vi "Adquisicion Sonido Continuo.vi"() -> ()   [LabVIEW 2023]
uses:
  <vilib>/sound2/lvsound2.llb/Sound Data Format.ctl
  <vilib>/sound2/lvsound2.llb/Sampling Mode.ctl
  <vilib>/sound2/lvsound2.llb/Sound Input Read (DBL).vi
  <vilib>/express/express analysis/Spectral/Block/exnSpectralBlock spectral measurements power poly.vi
  <vilib>/express/express analysis/Spectral/Block/exnSpectralBlock spectral measurements power array WFM.vi
  <vilib>/express/express analysis/Spectral/XNode/ExpressSpectralMeasurementsBlockNode.xnode
  <vilib>/measure/NI_MABase.lvlib
panel:
  in  "frequency":dbl=10.0 format="%0.2p"
  in  "signal type 2":T1(ring)
  in  "offset 2":dbl format="%0.2p"
  in  "phase 2":dbl format="%.2p"
  in  "amplitude 2":dbl=1.0 format="%0.2p"
  in  "signal type":T1(ring)
  in  "offset":dbl format="%0.2p"
  in  "phase":dbl format="%.2p"
  in  "amplitude":dbl=1.0 format="%0.2p"
  out "Max banda 2":i32
  out "Max banda 1":i32
  out "XY Graph":cluster{"Array":dbl[], "Array":dbl[]}(graph)
  out "Tamaño banda 2":i32
  out "Plano Y":dbl[](array[numeric])
  out "Tamaño banda 1":i32
  out "Plano X":dbl[](array[numeric])
  in  "banda 2":dbl
  in  "banda 1":dbl
  out "Tamaño Señal":i32
  out "Espectro Señal":cluster{"f0":dbl, "df":dbl, "magnitude":dbl[]}[](graph)
  in  "stop":bool
  in  "Tiempo de refresco":dbl
  out "Señal Adquirida":waveform(dbl)[](graph)
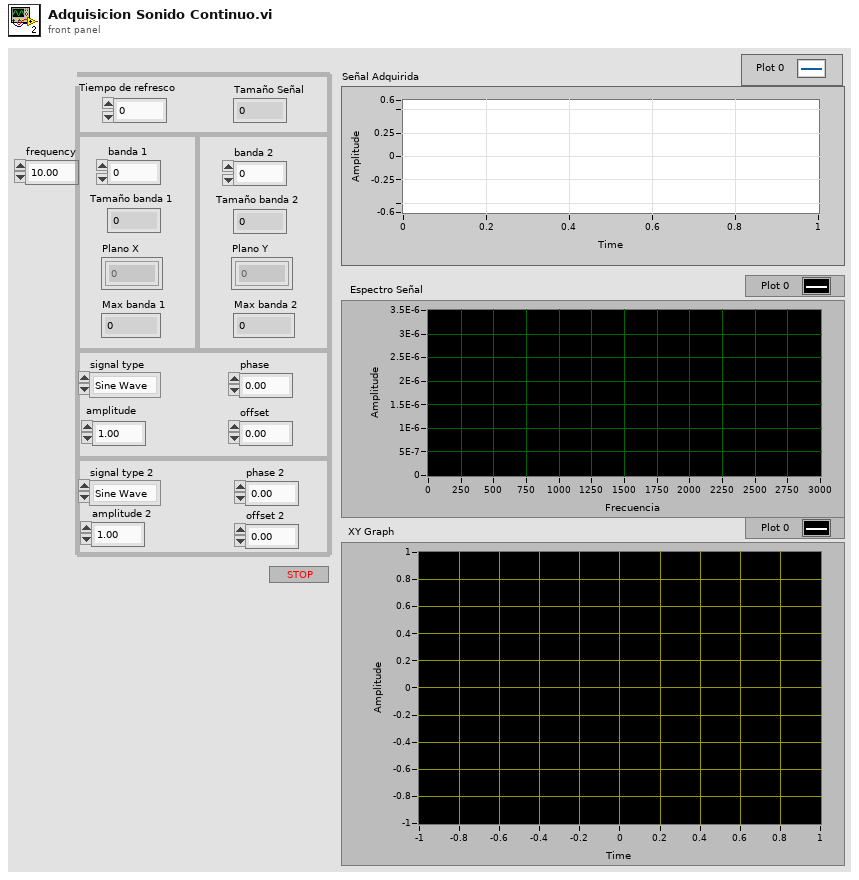
[diagram p1: front panel]
types:
  T1 = enum16{"Sine Wave", "Triangle Wave", "Square Wave", "Sawtooth Wave"}
  T2 = typedef "Sampling Mode.ctl" = i32
  T3 = typedef "Sound Data Format.ctl" = cluster{"sample rate (S/s)":dbl, "number of channels":i32, "bits per sample":i32}
  T4 = typedef "Sound Input Task ID.ctl" = u32
  T5 = cluster{"averaging mode":u16, "weighting mode":u16, "number of averages":u32}
  T6 = cluster{"dB On (F)":bool, "unwrap phase (F)":bool, "convert to degree (F)":bool}
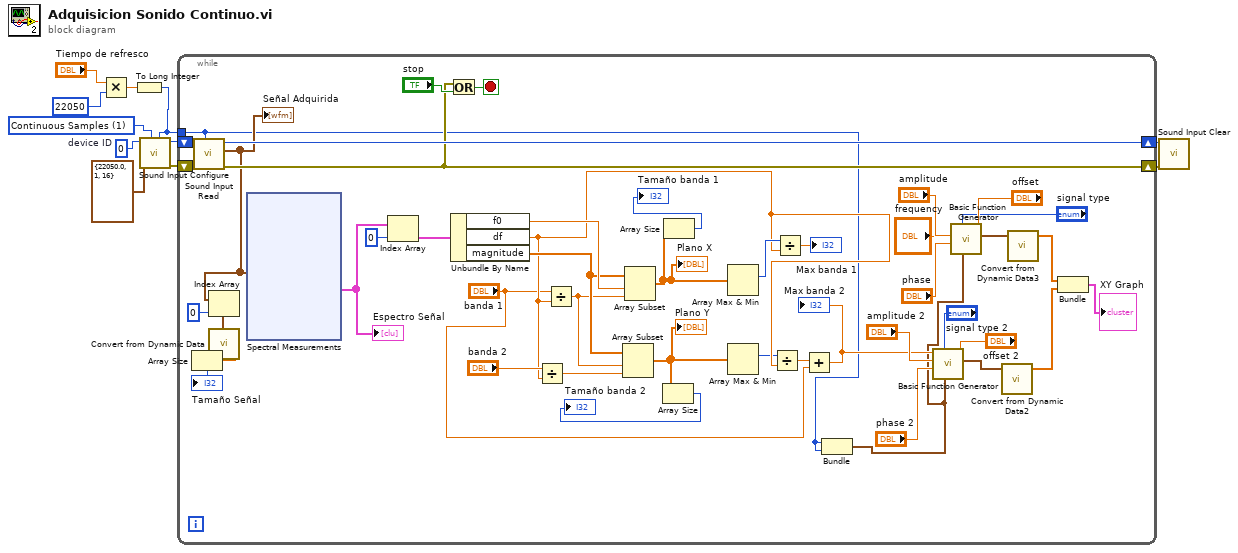
[diagram p0: block diagram]
diagram:
  w6 = u32 0  # device ID
  w10 = T2 1 items=["Finite Samples", "Continuous Samples"] ("sample mode")
  n1 = Multiply(x="Tiempo de refresco", y=22050 ("number of samples/ch")) -> (x*y=w5:dbl)
  n2 = To Long Integer(number=w5) -> (32bit integer=w7:i32)
  n3 = call <vilib>:"Sound Input Configure.vi"("number of samples/ch"=w7, "sample mode"=w10, "sound format"=T3 {"sample rate (S/s)"=22050.0, "number of channels"=1, "bits per sample"=16}, "device ID"=w6) -> ("error out"=w8:errorcluster, "task ID"=w9:T4)  [unwired: 6 in]
  n4 = while {
    tunnel: w7 -> [w12]
    shift-right: [w53] -> w3
    shift-left: w9 -> [w57]
    shift-right: [w52] -> w2
    shift-left: w8 -> [w56]
    stop <- w54 stop-if-true
    n5 = call-poly <vilib>:"Sound Input Read.vi"("number of samples/ch"=w12, "error in (no error)"=w56, "task ID"=w57) -> ("error out"=w52:errorcluster, "data"=w49:waveform(dbl)[], "task ID out"=w53:T4)  [unwired: 6 in]
    "Señal Adquirida" <- w49
    n6 = Index Array(array=w49, index=0) -> (element=w47:waveform(dbl))
    n7 = call "Convert from Dynamic Data"("Dynamic Data Type"=w47) -> ("Array"=w46:dbl[])  [unwired: 3 in]
    n8 = Array Size(array=w46) -> (size(s)=→"Tamaño Señal":i32)
    n9 = xnode "Spectral Measurements"("Signals"=w49) -> ("Power Spectrum"=w51:cluster{"f0":dbl, "df":dbl, "magnitude":dbl[]}[])  [unwired: 1 in, 1 out]
    "Espectro Señal" <- w51
    n10 = Index Array(array=w51, index=0) -> (element=w50:cluster{"f0":dbl, "df":dbl, "magnitude":dbl[]})
    n11 = Or(x=w52, y="stop") -> (x .or. y?=w54:bool)
    n12 = Unbundle By Name(w50) -> ("f0"=w44:dbl, "df"=w33:dbl, "magnitude"=w41:dbl[])
    n13 = Divide(x="banda 2", y=w33) -> (x/y=w42:dbl)
    n14 = Divide(x="banda 1", y=w33) -> (x/y=w36:dbl)
    n15 = Array Subset(array=w41, index=w36, length=w42) -> (w35:dbl[])
    "Plano Y" <- w35
    n16 = Array Subset(array=w41, index=w44, length=w36) -> (w38:dbl[])
    "Plano X" <- w38
    n17 = Array Size(array=w35) -> (size(s)=→"Tamaño banda 2":i32)
    n18 = Array Size(array=w38) -> (size(s)=→"Tamaño banda 1":i32)
    n19 = Array Max & Min(array=w38) -> (max index (indices)=w34:i32)  [unwired: 3 out]
    n20 = Array Max & Min(array=w35) -> (max index (indices)=w32:i32)  [unwired: 3 out]
    n21 = Divide(x=w32, y=w33) -> (x/y=w31:dbl)
    n22 = Divide(x=w34, y=w33) -> (x/y=→"Max banda 1":dbl)
    n23 = Add(x=w31, y="banda 1") -> (x+y=w20:dbl)
    "Max banda 2" <- w20
    n24 = Bundle(w12, w12) -> (w15:cluster{i32, i32})  [unwired: 1 in]
    n25 = call <vilib>:"Basic Function Generator.vi"("offset"="offset 2", "sampling info"=w15, "signal type"="signal type 2", "phase"="phase 2", "amplitude"="amplitude 2", "frequency"=w20) -> ("signal out"=w19:waveform(dbl))  [unwired: 3 in, 2 out]
    n26 = call <vilib>:"Basic Function Generator.vi"("offset"="offset", "sampling info"=w15, "signal type"="signal type", "phase"="phase", "amplitude"="amplitude", "frequency"="frequency") -> ("signal out"=w18:waveform(dbl))  [unwired: 3 in, 2 out]
    n27 = call "Convert from Dynamic Data2"("Dynamic Data Type"=w19) -> ("Array"=w17:dbl[])  [unwired: 3 in]
    n28 = call "Convert from Dynamic Data3"("Dynamic Data Type"=w18) -> ("Array"=w16:dbl[])  [unwired: 3 in]
    n29 = Bundle("Array"=w16, "Array"=w17) -> (→"XY Graph":cluster{"Array":dbl[], "Array":dbl[]})  [unwired: 1 in]
  }
  n30 = call <vilib>:"Sound Input Clear.vi"("error in (no error)"=w2, "task ID"=w3) -> ()  [unwired: 9 in, 1 out]
